vi "Pre Launch Init.vi"(11 "root_actor in":refnum<class "root_actor.lvclass">) -> (0 "error out":errorcluster, 3 "root_actor out":refnum<class "root_actor.lvclass">)   [LabVIEW 2025, in "root_actor.lvlib" / "root_actor.lvclass"]
doc: "(<B>Filename</B>: Actor Framework.lvlib:Actor.lvclass:Pre Launch Init.vi)\n\nDefines behavior that occurs after the Launch Nested Actor method is invoked but before the actor's Actor Core method begins running.\n\nBy default, this method does nothing. A descendant class may override it to define behavior."
uses:
  root_actor.lvclass
  DAQVoltage/DAQVoltage/DAQVoltage.lvclass
  Applications/National Instruments/LabVIEW 2025 64-bit/vi.lib/ActorFramework/Actor/Actor.lvclass
  command_parser/command_parser/command_parser.lvclass
  UDP_transmitter/UDP_transmitter/UDP_transmitter.lvclass
  UDP_receiver/UDP_receiver/UDP_receiver.lvclass
  root_actor.lvclass/root_actor.ctl
  <vilib>/ActorFramework/Actor/Actor.lvclass
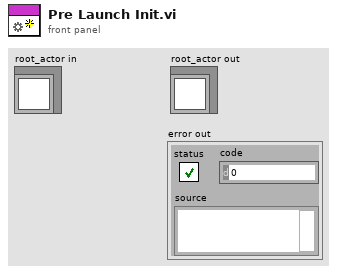
[diagram p1: front panel]
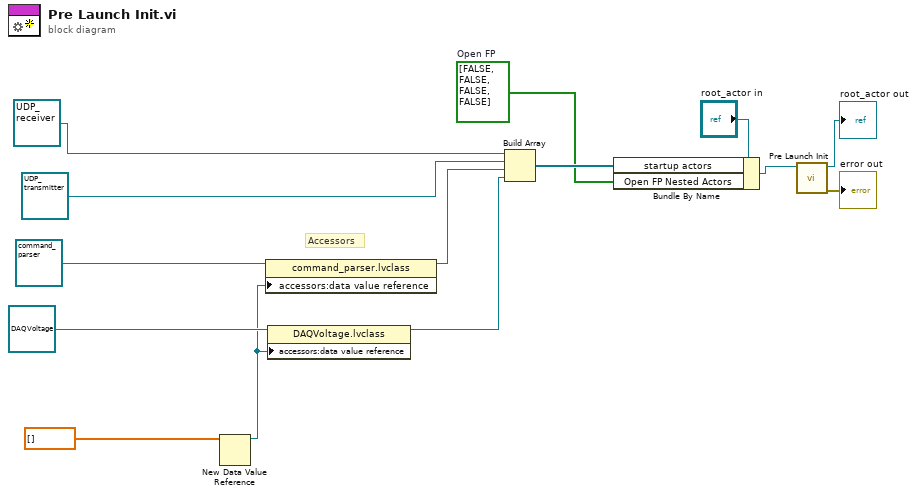
[diagram p0: block diagram]
diagram:
  w8 = bool[] [FALSE, FALSE, FALSE, FALSE]  # Open FP
  # "Accessors"
  n1 = New Data Value Reference(data value=dbl[] []) -> (data value reference=w3:refnum<data-value>)  [unwired: 1 in, 1 out]
  n2 = property class="command_parser.lvclass"(reference=refnum<class "command_parser.lvclass"> refnum ("command_parser.lvlib:command_parser.lvclass"), "accessors:data value reference"=w3) -> (reference out=w7:refnum<class "command_parser.lvclass">)  [unwired: 1 in, 1 out]
  n3 = property class="DAQVoltage.lvclass"(reference=refnum<class "DAQVoltage.lvclass"> refnum ("DAQVoltage.lvlib:DAQVoltage.lvclass"), "accessors:data value reference"=w3) -> (reference out=w5:refnum<class "DAQVoltage.lvclass">)  [unwired: 1 in, 1 out]
  n4 = Build Array(refnum<class "UDP_receiver.lvclass"> refnum ("UDP_receiver.lvlib:UDP_receiver.lvclass"), refnum<class "UDP_transmitter.lvclass"> refnum ("UDP_transmitter.lvlib:UDP_transmitter.lvclass"), w7, w5) -> (w10:refnum<class "Actor.lvclass">[])
  n5 = Bundle By Name(cluster="root_actor in", "startup actors"=w10, "Open FP Nested Actors"=w8) -> (w9:refnum<class "root_actor.lvclass">)
  n6 = call-parent "Pre Launch Init.vi"("Actor in"=w9) -> ("error out"=→"error out":errorcluster, "Actor out"=→"root_actor out":refnum<class "root_actor.lvclass">)  [unwired: 9 in]
